vi "Compose JSON String (JSON).vi"(8 "error in (no error)":errorcluster, 11 "Value":T1) -> (0 "error out":errorcluster, 3 "String":string)   [LabVIEW 2015, in "JSON.lvlib"]
uses:
  JSON.lvlib
  JSON Value.ctl
  Compose Data.ctl
  Value.ctl
  Value Type.ctl
  Name-Value Pair.ctl
  <vilib>/regexp/Match Regular Expression.xnode
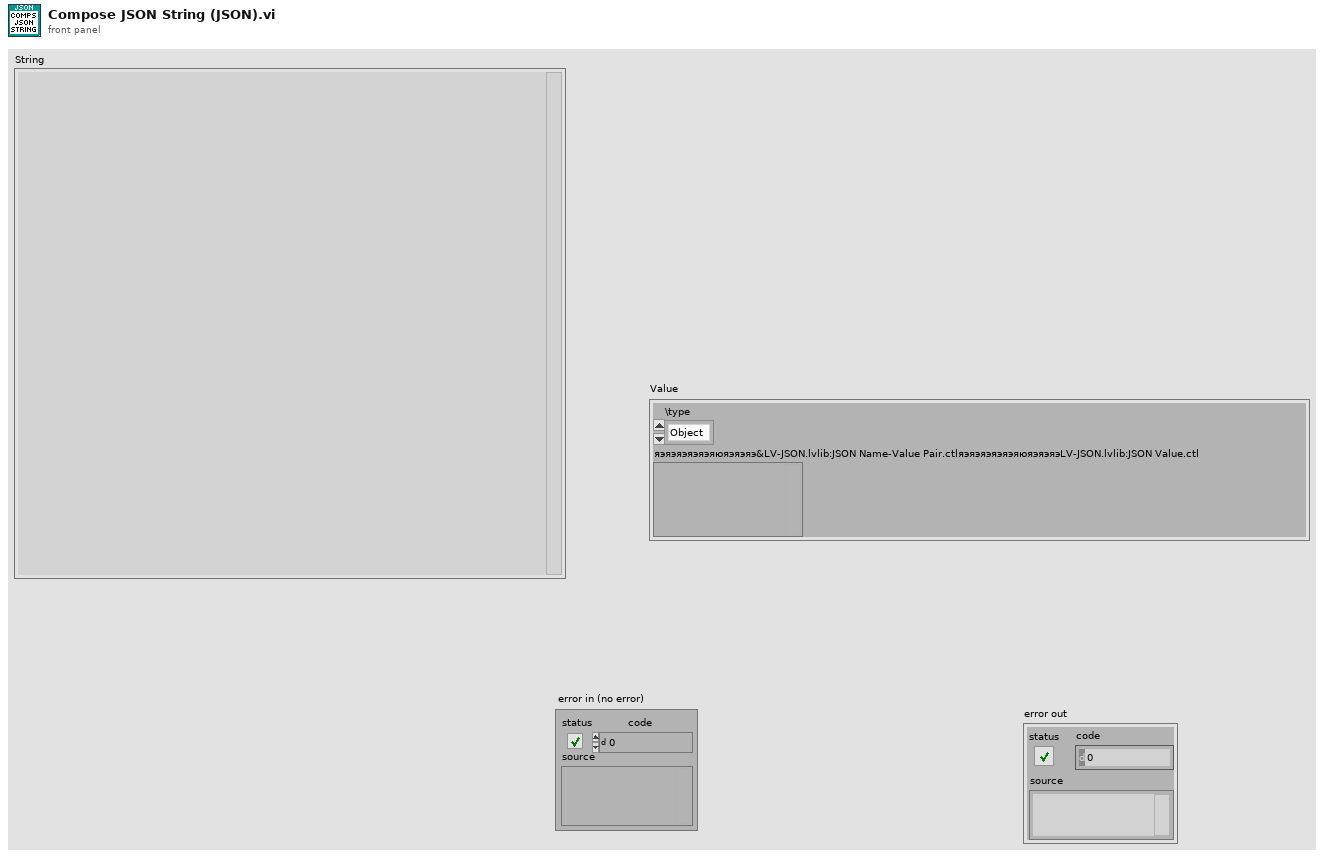
[diagram p1: front panel]
types:
  T1 = typedef "JSON.lvlib/JSON Value.ctl" = cluster{"\\type":enum16{"Object", "Array", "String", "Number", "Boolean", "Null"}, "яэяэяэяэяэяюяэяэяэ&LV-JSON.lvlib:JSON Name-Value Pair.ctlяэяэяэяэяэяюяэяэяэLV-JSON.lvlib:JSON Value.ctl":variant}
  T2 = typedef "JSON.lvlib/Compose Data.ctl" = cluster{"Value":T3, "Prepend":string, "Append":string}
  T3 = typedef "JSON.lvlib/Value.ctl" = cluster{"Type":T4, "Value":variant}
  T4 = typedef "JSON.lvlib/Value Type.ctl" = enum16{"Object", "Array", "String", "Number", "Boolean", "Null"}
  T5 = typedef "JSON.lvlib/Name-Value Pair.ctl" = cluster{"Name":string, "Value":T3}
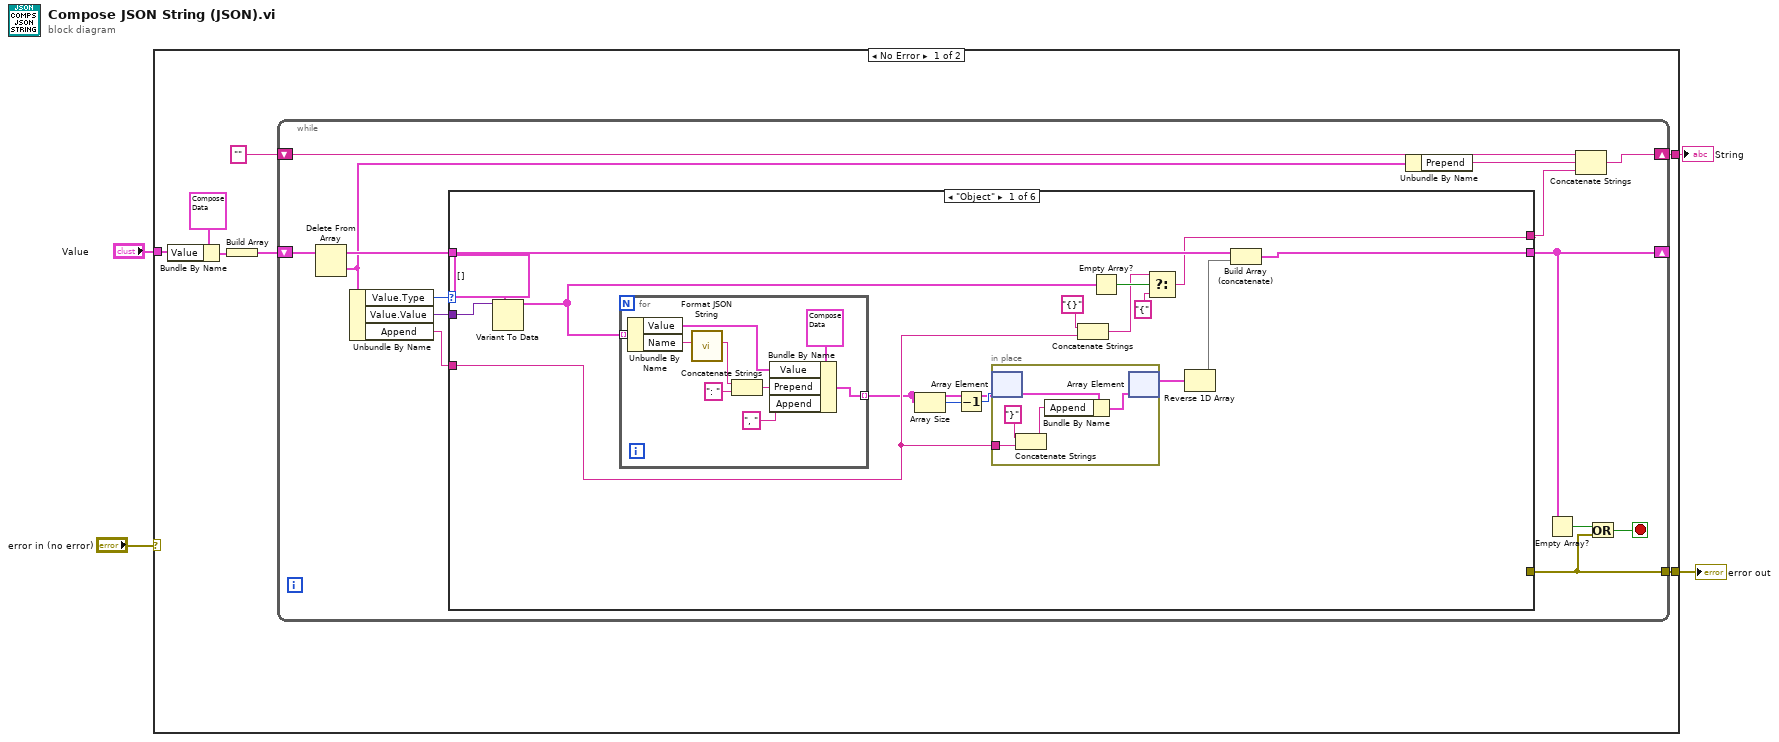
[diagram p0: block diagram]
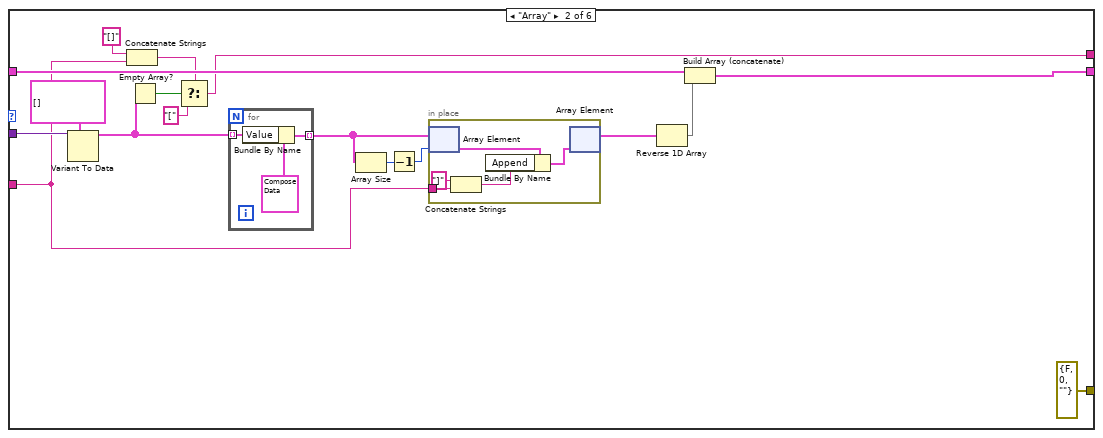
[diagram p2: hidden frame]
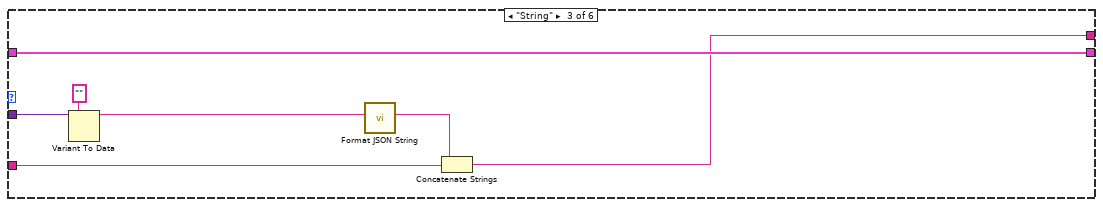
[diagram p3: hidden frame]
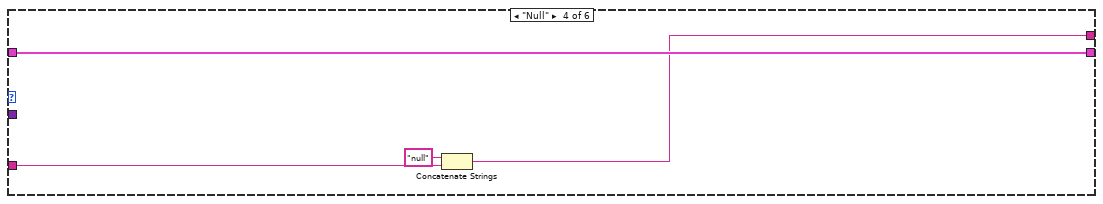
[diagram p4: hidden frame]
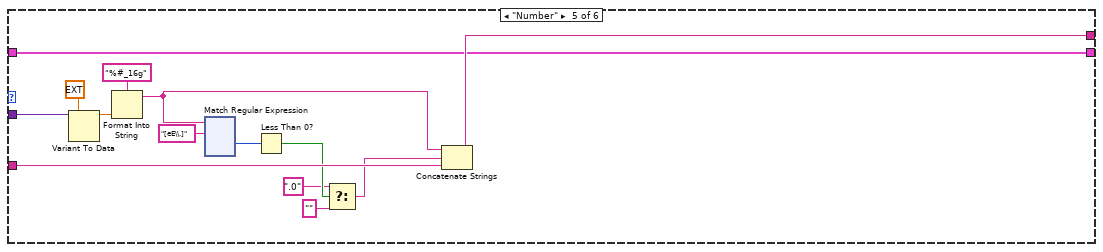
[diagram p5: hidden frame]
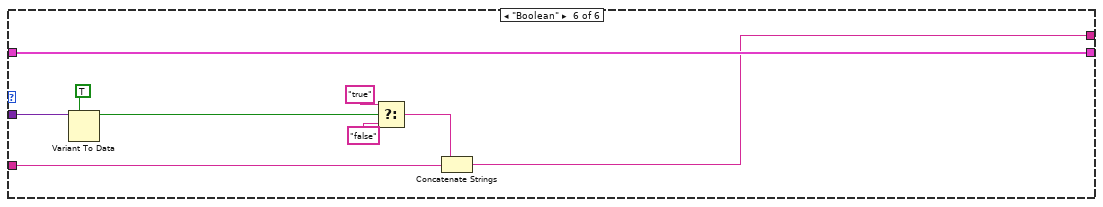
[diagram p6: hidden frame]
diagram:
  n1 = case shown="No Error" "error in (no error)" {
    selector: "error in (no error)" -> [_ w229]
    tunnel: "Value" -> [w8 _]
    tunnel: [w6 _] -> w3
    tunnel: [w5 w229] -> w1
    frame No Error {
      n2 = Bundle By Name(cluster=T2 {"Value"={"Type"=enum."Object", "Value"=variant}, "Prepend"="", "Append"=""}, "Value"=w8) -> (w7:T2)
      n3 = Build Array(w7) -> (w10:T2[])
      n4 = while {
        shift-right: [w18] -> w6
        shift-left: "" -> [w21]
        shift-right: [w19] -> _
        shift-left: w10 -> [w25]
        tunnel: [w12] -> w5
        stop <- w13 stop-if-true
        n5 = Delete From Array(array=w25) -> (deleted portion=w16:T2, array with subset deleted=w22:T2[])  [unwired: 2 in]
        n6 = Unbundle By Name(w16) -> ("Value.Type"=w24:T4, "Value.Value"=w23:variant, "Append"=w14:string)
        n7 = case shown="\"Object\"" w24 {
          tunnel: w23 -> [w39 w72 w86 _ w105 w228]
          tunnel: w22 -> [w41 w68 w87 w91 w100 w226]
          tunnel: [w40 w61 w87 w91 w100 w226] -> w19
          tunnel: [w35 w59 w81 w89 w102 w220] -> w17
          tunnel: w14 -> [w36 w62 w82 w90 w103 w227]
          tunnel: [_ errorcluster {"status"=FALSE, "code"=0, "source"=""} ("error constant") _ _ _ _] -> w12
          frame "Object" {
            n8 = Variant To Data(type=T5[] [], Variant=w39) -> (data=w37:T5[])  [unwired: 1 in, 1 out]
            n9 = for {
              tunnel: w37 -> [w55] mode=indexing
              tunnel: [w50] -> w32 mode=indexing
              n10 = Unbundle By Name(w55) -> ("Value"=w53:T3, "Name"=w48:string)
              n11 = call "Format JSON String.vi"("String"=w48) -> ("Formatted Basic String"=w47:string)  [unwired: 10 in]
              n12 = Concatenate Strings(w47, ": " ("string")) -> (w52:string)
              n13 = Bundle By Name(cluster=T2 {"Value"={"Type"=enum."Object", "Value"=variant}, "Prepend"="", "Append"=""}, "Value"=w53, "Prepend"=w52, "Append"=", ") -> (w50:T2)
            }
            n14 = Array Size(array=w32) -> (size(s)=w34:i32)
            n15 = Decrement(x=w34) -> (x-1=w33:i32)
            n16 = in-place {
              in-place-border: w36 -> [w42]
              n17 = in-place-array #1(w32, w33) -> (w46:T2)
              n18 = Concatenate Strings("}" ("Prepend"), w42) -> (w43:string)
              n19 = Bundle By Name(cluster=w46, "Append"=w43) -> (w45:T2)
              n20 = in-place-array #1(w45) -> (w29:T2[])  [unwired: 1 out]
            }
            n21 = Concatenate Strings("{}" ("Prepend"), w36) -> (w26:string)
            n22 = Empty Array?(array=w37) -> (empty?=w31:bool)
            n23 = Select(t=w26, s=w31, f="{" ("t")) -> (s? t:f=w35:string)
            n24 = Reverse 1D Array(array=w29) -> (reversed array=w28:T2[])
            n25 = Build Array (concatenate)(w41, w28) -> (w40:T2[])
          }
          frame "Array" {
            n26 = Variant To Data(type=T3[] [], Variant=w72) -> (data=w60:T3[])  [unwired: 1 in, 1 out]
            n27 = Concatenate Strings("[]", w62) -> (w63:string)
            n28 = Empty Array?(array=w60) -> (empty?=w65:bool)
            n29 = Select(t=w63, s=w65, f="[") -> (s? t:f=w59:string)
            n30 = for {
              tunnel: w60 -> [w80] mode=indexing
              tunnel: [w79] -> w70 mode=indexing
              n31 = Bundle By Name(cluster=T2 {"Value"={"Type"=enum."Object", "Value"=variant}, "Prepend"="", "Append"=", "}, "Value"=w80) -> (w79:T2)
            }
            n32 = Array Size(array=w70) -> (size(s)=w57:i32)
            n33 = Decrement(x=w57) -> (x-1=w56:i32)
            n34 = in-place {
              in-place-border: w62 -> [w73]
              n35 = in-place-array #2(w70, w56) -> (w77:T2)
              n36 = Concatenate Strings("]" ("string"), w73) -> (w75:string)
              n37 = Bundle By Name(cluster=w77, "Append"=w75) -> (w76:T2)
              n38 = in-place-array #2(w76) -> (w69:T2[])  [unwired: 1 out]
            }
            n39 = Reverse 1D Array(array=w69) -> (reversed array=w67:T2[])
            n40 = Build Array (concatenate)(w68, w67) -> (w61:T2[])
          }
          frame "String" {
            n41 = Variant To Data(type="", Variant=w86) -> (data=w84:string)  [unwired: 1 in, 1 out]
            n42 = call "Format JSON String.vi"("String"=w84) -> ("Formatted Basic String"=w83:string)  [unwired: 10 in]
            n43 = Concatenate Strings(w83, w82) -> (w81:string)
          }
          frame "Null" {
            n44 = Concatenate Strings("null" ("string"), w90) -> (w89:string)
          }
          frame "Number" {
            n45 = Variant To Data(type=ext 0.0, Variant=w105) -> (data=w101:ext)  [unwired: 1 in, 1 out]
            n46 = Format Into String(format string="%#_16g", w101) -> (resulting string=w95:string)  [unwired: 2 in, 1 out]
            n47 = xnode "Match Regular Expression"("input string"=w95, "regular expression"="[eE\\.]") -> ("offset past match"=w97:i32)  [unwired: 4 in, 4 out]
            n48 = Less Than 0?(x=w97) -> (x < 0?=w96:bool)
            n49 = Select(t=".0", s=w96, f="") -> (s? t:f=w92:string)
            n50 = Concatenate Strings(w95, w92, w103) -> (w102:string)
          }
          frame "Boolean" {
            n51 = Variant To Data(type=TRUE, Variant=w228) -> (data=w224:bool)  [unwired: 1 in, 1 out]
            n52 = Select(t="true", s=w224, f="false") -> (s? t:f=w221:string)
            n53 = Concatenate Strings(w221, w227) -> (w220:string)
          }
        }
        n54 = Unbundle By Name(w16) -> ("Prepend"=w15:string)
        n55 = Empty Array?(array=w19) -> (empty?=w20:bool)
        n56 = Concatenate Strings(w21, w15, w17) -> (w18:string)
        n57 = Or(x=w20, y=w12) -> (x .or. y?=w13:bool)
      }
    }
    frame Error {
    }
  }
  "String" <- w3
  "error out" <- w1
